vi "ssh_example.vi"() -> ()   [LabVIEW 2024]
uses:
  <vilib>/net/SSH/Client/OpenSSH/OpenSSH Client.lvclass
  C:/Program Files (x86)/National Instruments/LabVIEW 2024/vi.lib/net/SSH/Client/Generic/Generic Client.lvclass
  <vilib>/net/SSH/Client/Generic/Generic Client.lvclass/Generic Client.ctl
  <vilib>/net/SSH/Client/Generic/Write user_host.vi
  <vilib>/net/SSH/Client/Generic/Write trust on first use.vi
  <vilib>/net/SSH/NI_SSH.lvlib
panel:
  in  "error in (no error)":errorcluster
  out "error out":errorcluster
  out "standard error":string
  out "standard output":string
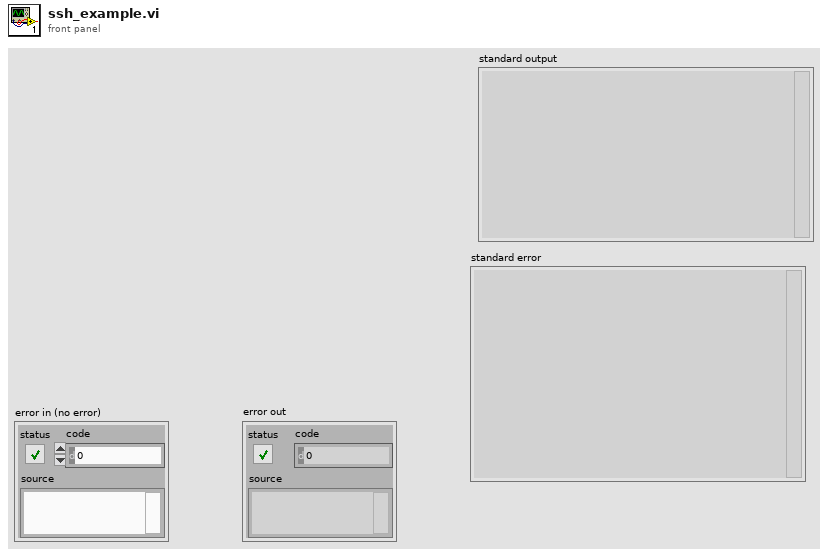
[diagram p1: front panel]
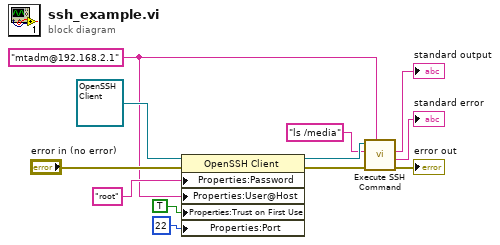
[diagram p0: block diagram]
diagram:
  w1 = "mtadm@192.168.2.1" ("User@Host")
  n1 = property class="OpenSSH Client"(reference=refnum<class "OpenSSH Client.lvclass"> refnum ("NI_SSH.lvlib:OpenSSH Client"), error in="error in (no error)", "Properties:Password"="root" ("Password"), "Properties:User@Host"=w1, "Properties:Trust on First Use"=TRUE ("Trust on First Use"), "Properties:Port"=u16 22 ("Port")) -> (reference out=w11:refnum<class "OpenSSH Client.lvclass">, error out=w10:errorcluster)
  n2 = call <vilib>:"Execute SSH Command.vi"("user@host"=w1, "error in (no error)"=w10, "command line"="ls /media", "session in"=w11) -> ("error out"=→"error out":errorcluster, "standard error"=→"standard error":string, "standard output"=→"standard output":string)  [unwired: 3 in, 2 out]
